vi "Pressure Mode.vi"(7 "Set? (F:Read)":bool, 8 "Error In":errorcluster, 9 "Pressure Mode (F:Off))":bool, 11 "VISA resource name":refnum<visa-resource-name>) -> (0 "Error Out":errorcluster, 1 "Pressure Mode":bool, 3 "dup VISA resource name":refnum<visa-resource-name>)   [LabVIEW 2016, in "MGC647C.lvlib"]
doc: "Read/Set pressure mode."
uses:
  MGC647C.lvlib
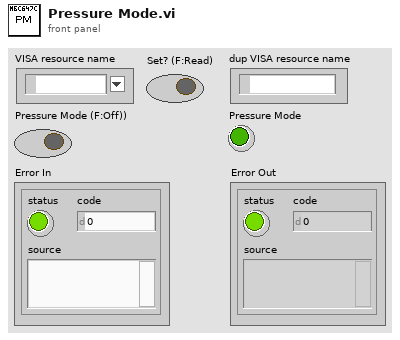
[diagram p1: front panel]
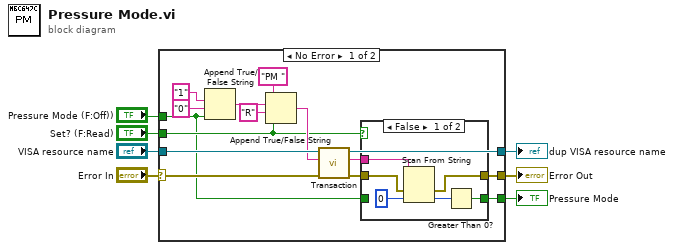
[diagram p0: block diagram]
diagram:
  n1 = case shown="No Error" "Error In" {
    selector: "Error In" -> [w14 w32]
    tunnel: "VISA resource name" -> [w22 w31]
    tunnel: [w21 w31] -> w6
    tunnel: [w20 w32] -> w5
    tunnel: "Set? (F:Read)" -> [w9 _]
    tunnel: [w13 _] -> w2
    tunnel: "Pressure Mode (F:Off))" -> [w8 _]
    frame No Error {
      n2 = Append True/False String(1:w8, 2:"0" ("false string"), 3:"1" ("true string")) -> (0:w12:string)  [unwired: 1 in]
      n3 = Append True/False String(1:w9, 2:"R" ("false string"), 3:w12, 4:"PM " ("string (\"\")")) -> (0:w15:string)
      n4 = call "Transaction.vi"("Error In"=w14, "Command"=w15, "VISA resource name"=w22) -> ("Error Out"=w16:errorcluster, "Response"=w17:string, "dup VISA resource name"=w21:refnum<visa-resource-name>)  [unwired: 6 in]
      n5 = case shown="False" w9 {
        tunnel: [w28 w30] -> w20
        tunnel: w17 -> [w26 _]
        tunnel: w16 -> [w25 w30]
        tunnel: [w23 w29] -> w13
        tunnel: w8 -> [_ w29]
        frame False {
          n6 = Scan From String(input string=w26, error in=w25, default 1=0) -> (error out=w28:errorcluster, output 1=w27:i32)  [unwired: 2 in, 2 out]
          n7 = Greater Than 0?(x=w27) -> (x > 0?=w23:bool)
        }
        frame True {
        }
      }
    }
    frame Error {
    }
  }
  "dup VISA resource name" <- w6
  "Error Out" <- w5
  "Pressure Mode" <- w2
